vi "Json_Data_ERDS_Always_Show.vi"(0 "ERD Output":cluster{"ERD Number":u16, "Data":string}, 2 "Json File Path":path, 11 "error in":errorcluster) -> (4 "ERD Output 2":T1 {"ERD Number" format="%.0x"}, 15 "error out":errorcluster)   [LabVIEW 2021]
uses:
  Common/LabVIEW GEA2 Toolkit/GEA3/type defs/ERD Read Data Out.ctl
  <vilib>/JDP Science/JSONtext/String Subset.vi
  <vilib>/JDP Science/JSONtext/support/Strip Quotes and Unescape.vi
  <vilib>/JDP Science/JSONtext/support/Unescape JSON string.vi
  <vilib>/JDP Science/JSONtext/Parsing/Parse Full Path or Item Name.vi
  <vilib>/JDP Science/JSONtext/Offset/Find Item Locations by Path.vi
  <vilib>/JDP Science/JSONtext/JSONtext.lvlib
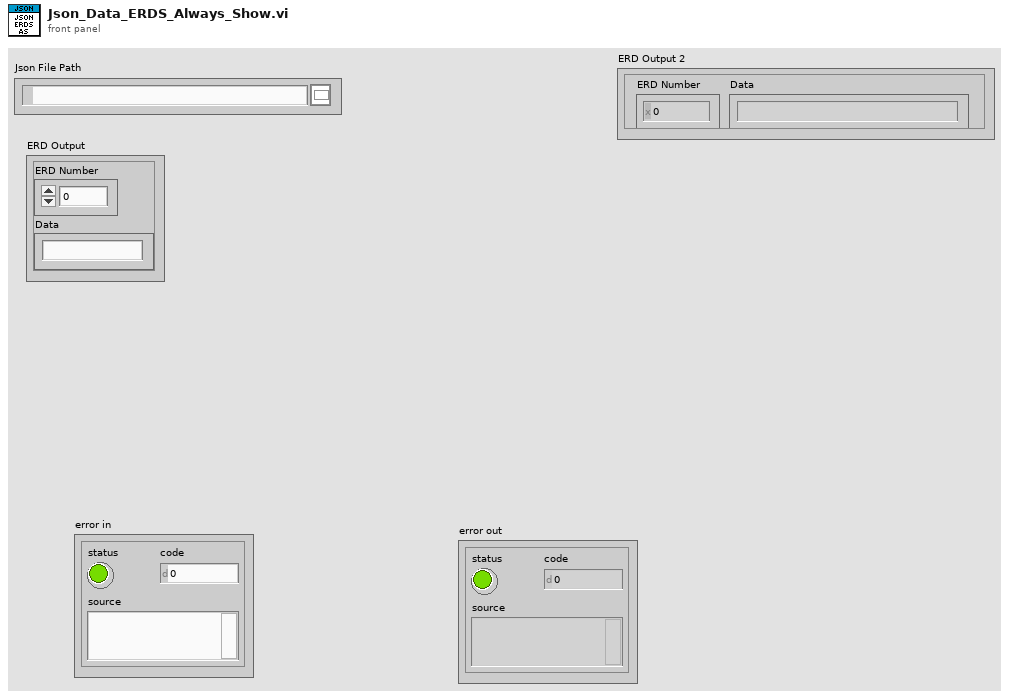
[diagram p1: front panel]
types:
  T1 = typedef "ERD Read Data Out.ctl" = cluster{"ERD Number":u16, "Data":string}
  T2 = enum16{"open", "replace", "create", "open or create", "replace or create", "replace or create with confirmation"}
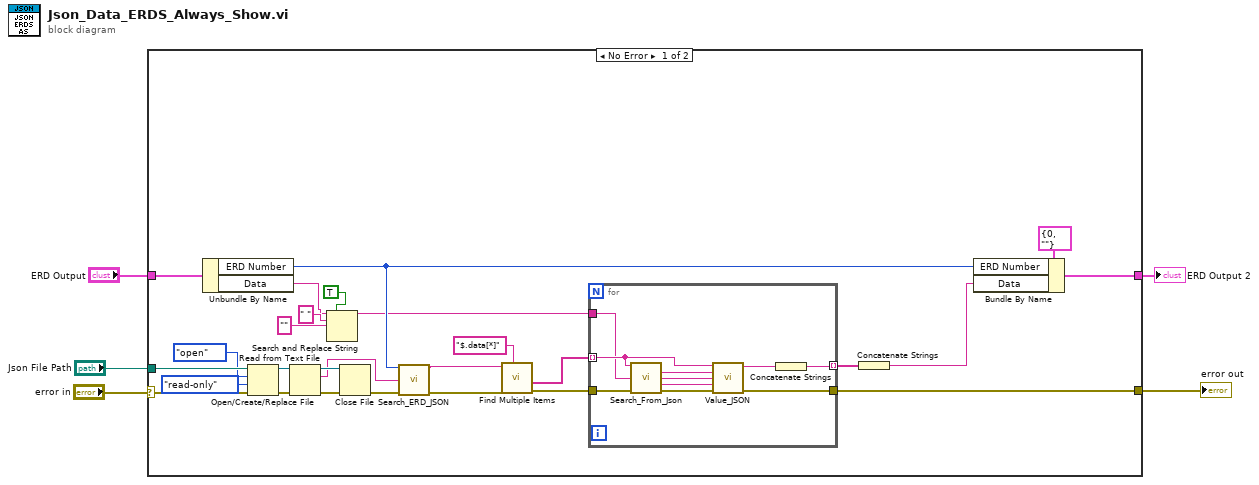
[diagram p0: block diagram]
diagram:
  n1 = case shown="No Error" "error in" {
    selector: "error in" -> [w25 w43]
    tunnel: [w19 w43] -> w4
    tunnel: "Json File Path" -> [w28 _]
    tunnel: [w8 _] -> w1
    tunnel: "ERD Output" -> [w10 _]
    frame No Error {
      n2 = Unbundle By Name(w10) -> ("ERD Number"=w16:u16, "Data"=w11:string)
      n3 = Open/Create/Replace File(file path (use dialog)=w28, error in=w25, operation (0:open)=T2."open", access (0:read/write)=enum16{"read/write", "read-only", "write-only"}."read-only") -> (refnum out=w30:refnum<file>, error out=w32:errorcluster)  [unwired: 2 in, 1 out]
      n4 = Read from Text File(file (use dialog)=w30, error in=w32) -> (refnum out=w29:refnum<file>, text=w20:string, error out=w31:errorcluster)  [unwired: 2 in, 1 out]
      n5 = Search and Replace String(replace all?=TRUE ("replace all? (F)"), input string=w11, search string=" ", replace string="" ("replace string (\"\")")) -> (result string=w12:string)  [unwired: 4 in, 3 out]
      n6 = Close File(refnum=w29, error in=w31) -> (error out=w21:errorcluster)  [unwired: 1 out]
      n7 = call "Search_ERD_JSON.vi"("ERD Number"=w16, "JSON Text"=w20, "error in"=w21) -> ("ERD"=w23:string, "error out"=w24:errorcluster)  [unwired: 11 in]
      n8 = call <vilib>:"Find Multiple Items.vi"("$Path or Item Name"="$.data[*]", "error in (no error)"=w24, "JSON"=w23) -> ("error out"=w22:errorcluster, "<JSON>"=w26:string[])  [unwired: 5 in, 2 out]
      n9 = for {
        tunnel: w26 -> [w42] mode=indexing
        tunnel: [w37] -> w19
        tunnel: w22 -> [w36]
        tunnel: w12 -> [w35]
        tunnel: [w34] -> w7 mode=indexing
        n10 = call "Search_From_Json.vi"("Data JSON"=w42, "ERD"=w35, "error in"=w36) -> ("Type"=w41:string, "Size data"=w40:string, "Hexa"=w39:string, "error IO"=w38:errorcluster)  [unwired: 8 in, 1 out]
        n11 = call "Value_JSON.vi"("Data JSON"=w42, "Type"=w41, "Size data"=w40, "Hexa"=w39, "error in"=w38) -> ("Value_string"=w33:string, "error IO"=w37:errorcluster)  [unwired: 8 in, 1 out]
        n12 = Concatenate Strings(w33) -> (w34:string)
      }
      n13 = Concatenate Strings(w7) -> (w6:string)
      n14 = Bundle By Name(cluster=T1 {"ERD Number"=0, "Data"=""} ("ERD Output"), "ERD Number"=w16, "Data"=w6) -> (w8:T1)
    }
    frame Error {
    }
  }
  "error out" <- w4
  "ERD Output 2" <- w1
